vi "controlRtOutTriggerConfig.vi"(7 "Set":bool, 8 "error in":errorcluster, 9 "Trigger Config":T1, 10 "axis in":u8, 11 "connection ID":i32) -> (0 "error out":errorcluster, 1 "Trigger Config out":T1, 2 "axis out":u8, 3 "connection ID":i32)   [LabVIEW 2016]
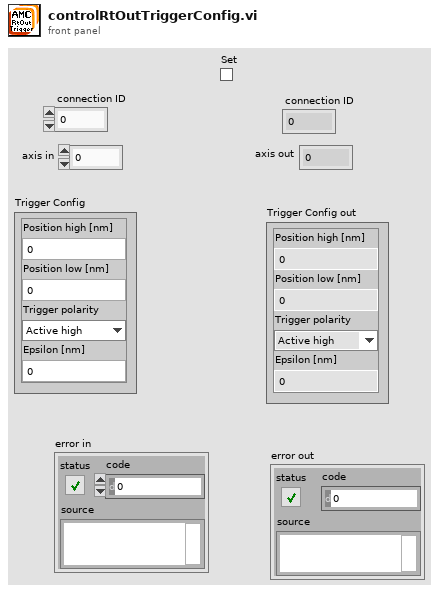
[diagram p1: front panel]
types:
  T1 = cluster{"Position high [nm]":i32, "Position low [nm]":i32, "Trigger polarity":enum16{"Active high", "Active low"}, "Epsilon [nm]":i32}
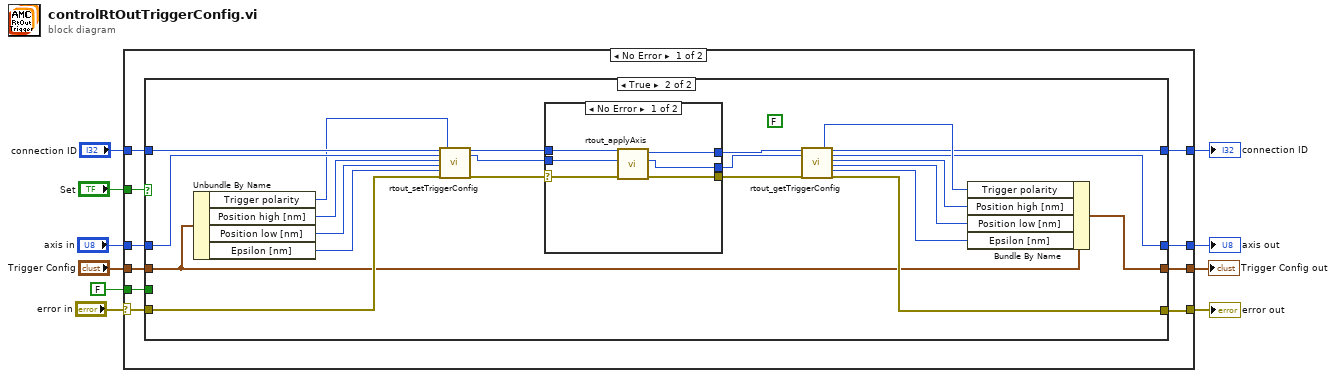
[diagram p0: block diagram]
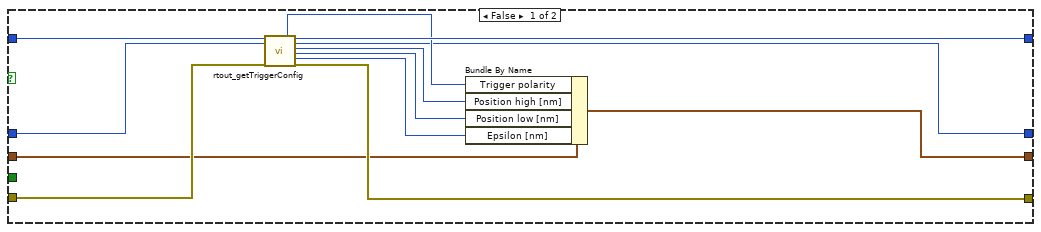
[diagram p2: hidden frame]
diagram:
  n1 = case shown="No Error" "error in" {
    selector: "error in" -> [w16 w67]
    tunnel: "axis in" -> [w18 w66]
    tunnel: [w17 w67] -> w9
    tunnel: [w14 w66] -> w8
    tunnel: "Set" -> [w19 _]
    tunnel: [w15 w65] -> w6
    tunnel: "connection ID" -> [w20 w65]
    tunnel: FALSE ("tempvalue") -> [w13 _]
    tunnel: "Trigger Config" -> [w12 w64]
    tunnel: [w11 w64] -> w1
    frame No Error {
      n2 = case shown="True" w19 {
        tunnel: w20 -> [w32 w54]
        tunnel: w18 -> [w28 w49]
        tunnel: [w29 w36] -> w17
        tunnel: w16 -> [w30 w52]
        tunnel: [w31 w38] -> w15
        tunnel: [w21 w37] -> w14
        tunnel: w13 -> [_ _]
        tunnel: w12 -> [w27 w34]
        tunnel: [w22 w35] -> w11
        frame False {
          n3 = call "rtout_getTriggerConfig.vi"("connection ID"=w32, "axis"=w28, "error in"=w30) -> ("polarity"=w26:i32, "connection ID"=w31:i32, "axis_out"=w21:i32, "higher"=w25:i32, "lower"=w24:i32, "epsilon"=w23:i32, "error out"=w29:errorcluster)  [unwired: 10 in]
          n4 = Bundle By Name(cluster=w27, "Trigger polarity"=w26, "Position high [nm]"=w25, "Position low [nm]"=w24, "Epsilon [nm]"=w23) -> (w22:T1)
        }
        frame True {
          (unwired) FALSE ("tempvalue")
          n5 = Unbundle By Name(w34) -> ("Trigger polarity"=w48:enum16{"Active high", "Active low"}, "Position high [nm]"=w47:i32, "Position low [nm]"=w46:i32, "Epsilon [nm]"=w45:i32)
          n6 = call "rtout_setTriggerConfig.vi"("connection ID"=w54, "axis"=w49, "higher"=w47, "lower"=w46, "epsilon"=w45, "error in"=w52, "polarity"=w48) -> ("connection ID"=w53:i32, "axis_out"=w50:i32, "error out"=w51:errorcluster)  [unwired: 10 in]
          n7 = case shown="No Error" w51 {
            selector: w51 -> [w59 w63]
            tunnel: [w58 w63] -> w39
            tunnel: w53 -> [w60 w61]
            tunnel: [w57 w61] -> w41
            tunnel: w50 -> [w56 w62]
            tunnel: [w55 w62] -> w40
            frame No Error {
              n8 = call "rtout_applyAxis.vi"("error in"=w59, "axis"=w56, "connection ID"=w60) -> ("error out"=w58:errorcluster, "axis_out"=w55:i32, "connection ID"=w57:i32)  [unwired: 6 in]
            }
            frame Error {
            }
          }
          n9 = call "rtout_getTriggerConfig.vi"("connection ID"=w41, "axis"=w40, "error in"=w39) -> ("polarity"=w44:i32, "connection ID"=w38:i32, "axis_out"=w37:i32, "higher"=w43:i32, "lower"=w42:i32, "epsilon"=w33:i32, "error out"=w36:errorcluster)  [unwired: 10 in]
          n10 = Bundle By Name(cluster=w34, "Trigger polarity"=w44, "Position high [nm]"=w43, "Position low [nm]"=w42, "Epsilon [nm]"=w33) -> (w35:T1)
        }
      }
    }
    frame Error {
    }
  }
  "error out" <- w9
  "axis out" <- w8
  "connection ID" <- w6
  "Trigger Config out" <- w1
